vi "Tool - Check Timeout.vi"(11 "error in (no error)":errorcluster, 12 "i":i32, 13 "Timeout, ms (10000)":i32=10000) -> (14 "Timeout?":bool, 15 "error out":errorcluster)   [LabVIEW 2012, in "REx.lvlib" / "Local Listener Session.lvclass"]
uses:
  Local Listener Session.lvclass
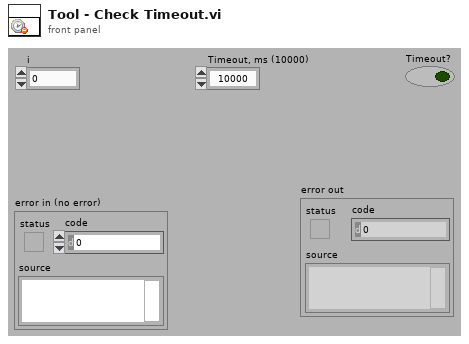
[diagram p1: front panel]
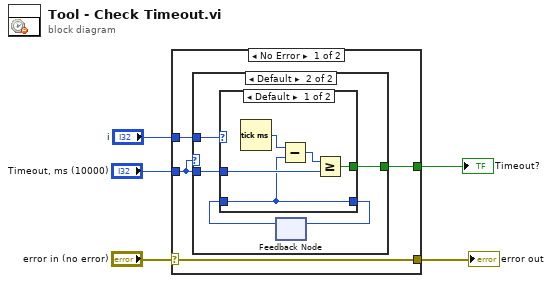
[diagram p0: block diagram]
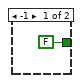
[diagram p2: hidden frame]
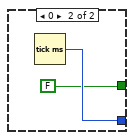
[diagram p3: hidden frame]
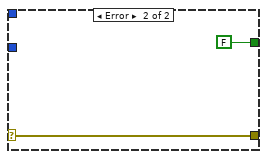
[diagram p4: hidden frame]
diagram:
  n1 = case shown="No Error" "error in (no error)" {
    selector: "error in (no error)" -> [w7 w24]
    tunnel: "i" -> [w9 _]
    tunnel: [w8 FALSE] -> w4
    tunnel: "Timeout, ms (10000)" -> [w6 _]
    tunnel: [w7 w24] -> w1
    frame No Error {
      n2 = case shown="Default" w6 {
        tunnel: w9 -> [_ w15]
        tunnel: [FALSE w12] -> w8
        tunnel: w6 -> [_ w11]
        frame -1 {
        }
        frame Default {
          n3 = feedback #1() -> (w13:u32)  [unwired: 1 in]
          n4 = case shown="Default" w15 {
            tunnel: [w16 w22] -> w14
            tunnel: [w19 FALSE] -> w12
            tunnel: w11 -> [w17 _]
            tunnel: w13 -> [w16 _]
            frame Default {
              n5 = Tick Count (ms)() -> (millisecond timer value=w20:u32)
              n6 = Subtract(x=w20, y=w16) -> (x-y=w18:u32)
              n7 = Greater Or Equal?(x=w18, y=w17) -> (x >= y?=w19:bool)
            }
            frame 0 {
              n8 = Tick Count (ms)() -> (millisecond timer value=w22:u32)
            }
          }
          n9 = feedback-in #1(w14) -> ()
        }
      }
    }
    frame Error {
    }
  }
  "Timeout?" <- w4
  "error out" <- w1
